vi "Path.vi"() -> ()   [LabVIEW 2014]
panel:
  out "Path":path
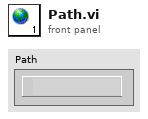
[diagram p1: front panel]
diagram:
